vi "Conditionally Connect Wire.vi"(8 "error in (no error)":errorcluster, 10 "Wire Source":refnum<vi>, 11 "Terminal in":refnum<vi>) -> (0 "error out":errorcluster, 3 "Terminal out":refnum<vi>)   [LabVIEW 2015, in "Scripting.lvlib"]
uses:
  Scripting.lvlib
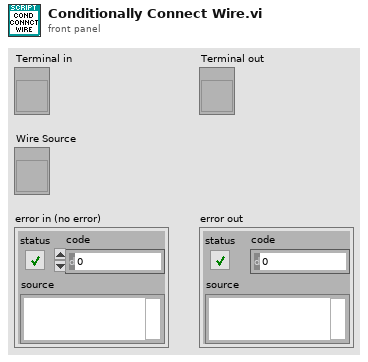
[diagram p1: front panel]
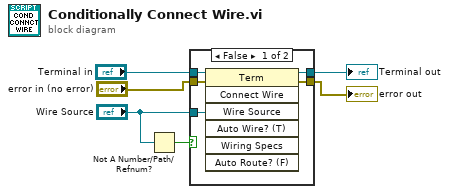
[diagram p0: block diagram]
diagram:
  n1 = Not A Number/Path/Refnum?(number/path/refnum="Wire Source") -> (NaN/Path/Refnum?=w4:bool)
  n2 = case shown="False" w4 {
    tunnel: "Terminal in" -> [w11 w12]
    tunnel: "Wire Source" -> [w10 _]
    tunnel: "error in (no error)" -> [w9 w13]
    tunnel: [w8 w13] -> w3
    tunnel: [w7 w12] -> w6
    frame False {
      n3 = invoke class="Term" method="Connect Wire"(reference=w11, error in=w9, "Wire Source"=w10) -> (reference out=w7:refnum<vi>, error out=w8:errorcluster)  [unwired: 4 in, 5 out]
    }
    frame True {
    }
  }
  "Terminal out" <- w6
  "error out" <- w3
